vi "enableZeroCorr.vi"(8 "error in (no error)":errorcluster, 10 "Enable Zero Correct (T: Enable)":bool, 11 "Electrometer in":refnum<class "Electrometer.lvclass">) -> (0 "error out":errorcluster, 3 "Electrometer out":refnum<class "Electrometer.lvclass">)   [LabVIEW 2016, in "Electrometer.lvclass"]
uses:
  Electrometer.lvclass
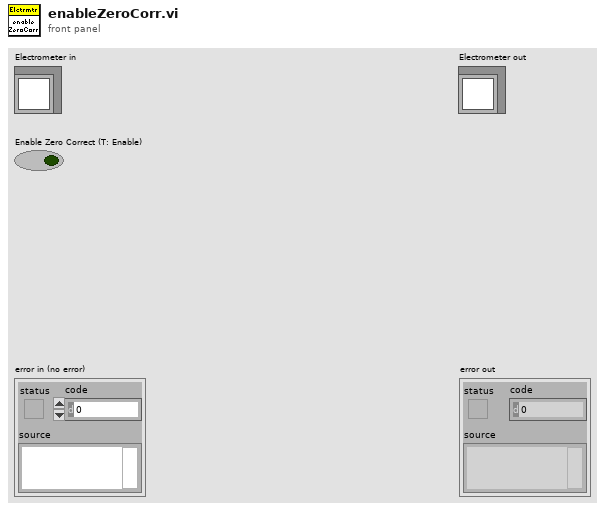
[diagram p1: front panel]
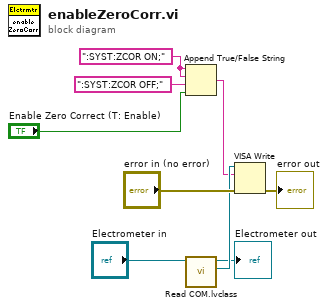
[diagram p0: block diagram]
diagram:
  w4 = ":SYST:ZCOR ON;"
  n1 = Append True/False String(1:"Enable Zero Correct (T: Enable)", 2:":SYST:ZCOR OFF;", 3:w4, 4:w4) -> (0:w1:string)
  n2 = call "Read COM.lvclass.vi"("Electrometer in"="Electrometer in") -> ("VISA"=w7:refnum<visa-resource-name>, "Electrometer out"=→"Electrometer out":refnum<class "Electrometer.lvclass">)  [unwired: 8 in, 1 out]
  n3 = VISA Write(VISA resource name=w7, write buffer=w1, error in (no error)="error in (no error)") -> (error out=→"error out":errorcluster)  [unwired: 2 out]
